vi "updateNVYPartsSerialNo.vi"() -> ()   [LabVIEW 2012]
uses:
  <vilib>/addons/database/Connection.llb/DB Tools Open Connec (Path).vi
  <vilib>/addons/database/Connection.llb/Conn Execute.vi
  <vilib>/addons/database/Recordset.llb/Rec Fetch String Data (R).vi
  <vilib>/addons/database/Recordset.llb/Rec Destroy - Connection.vi
  <vilib>/addons/database/Recordset.llb/Rec Fetch Recordset Data (R).vi
  <vilib>/addons/database/_DB Variant To Data/Database Variant To Data.xnode
  <vilib>/addons/database/NI_Database_API.lvlib
panel:
  out "date/time string 5":string
  out "data 10":string
  out "s? t:f 5":i32
  out "recordset data 5":variant[][](array[variant])
  out "error out 8":errorcluster
  out "error out 7":errorcluster
  out "data 9":string
  out "concatenated string 5":string
  out "x+y 5":i32
  out "date/time string 4":string
  out "data 8":string
  out "s? t:f 4":i32
  out "recordset data 4":variant[][](array[variant])
  out "error out 6":errorcluster
  out "error out 5":errorcluster
  out "data 7":string
  out "concatenated string 4":string
  out "x+y 4":i32
  out "error out 4":errorcluster
  out "date/time string 3":string
  out "data 6":string
  out "s? t:f 3":i32
  out "recordset data 3":variant[][](array[variant])
  out "error out 3":errorcluster
  out "data 5":string
  out "concatenated string 3":string
  out "x+y 3":i32
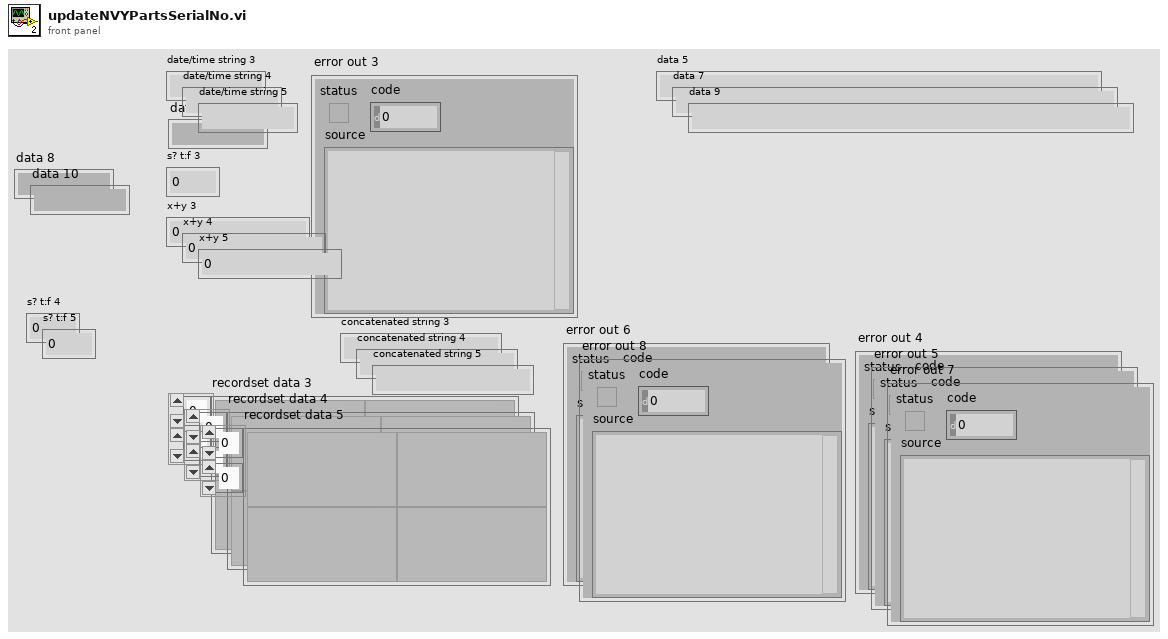
[diagram p1: front panel]
types:
  T1 = typedef "NI_Database_API.lvlib/Conn ObjectReference.ctl" = refnum<k1>
  T2 = typedef "NI_Database_API.lvlib/Rec ObjectReference.ctl" = refnum<k1>
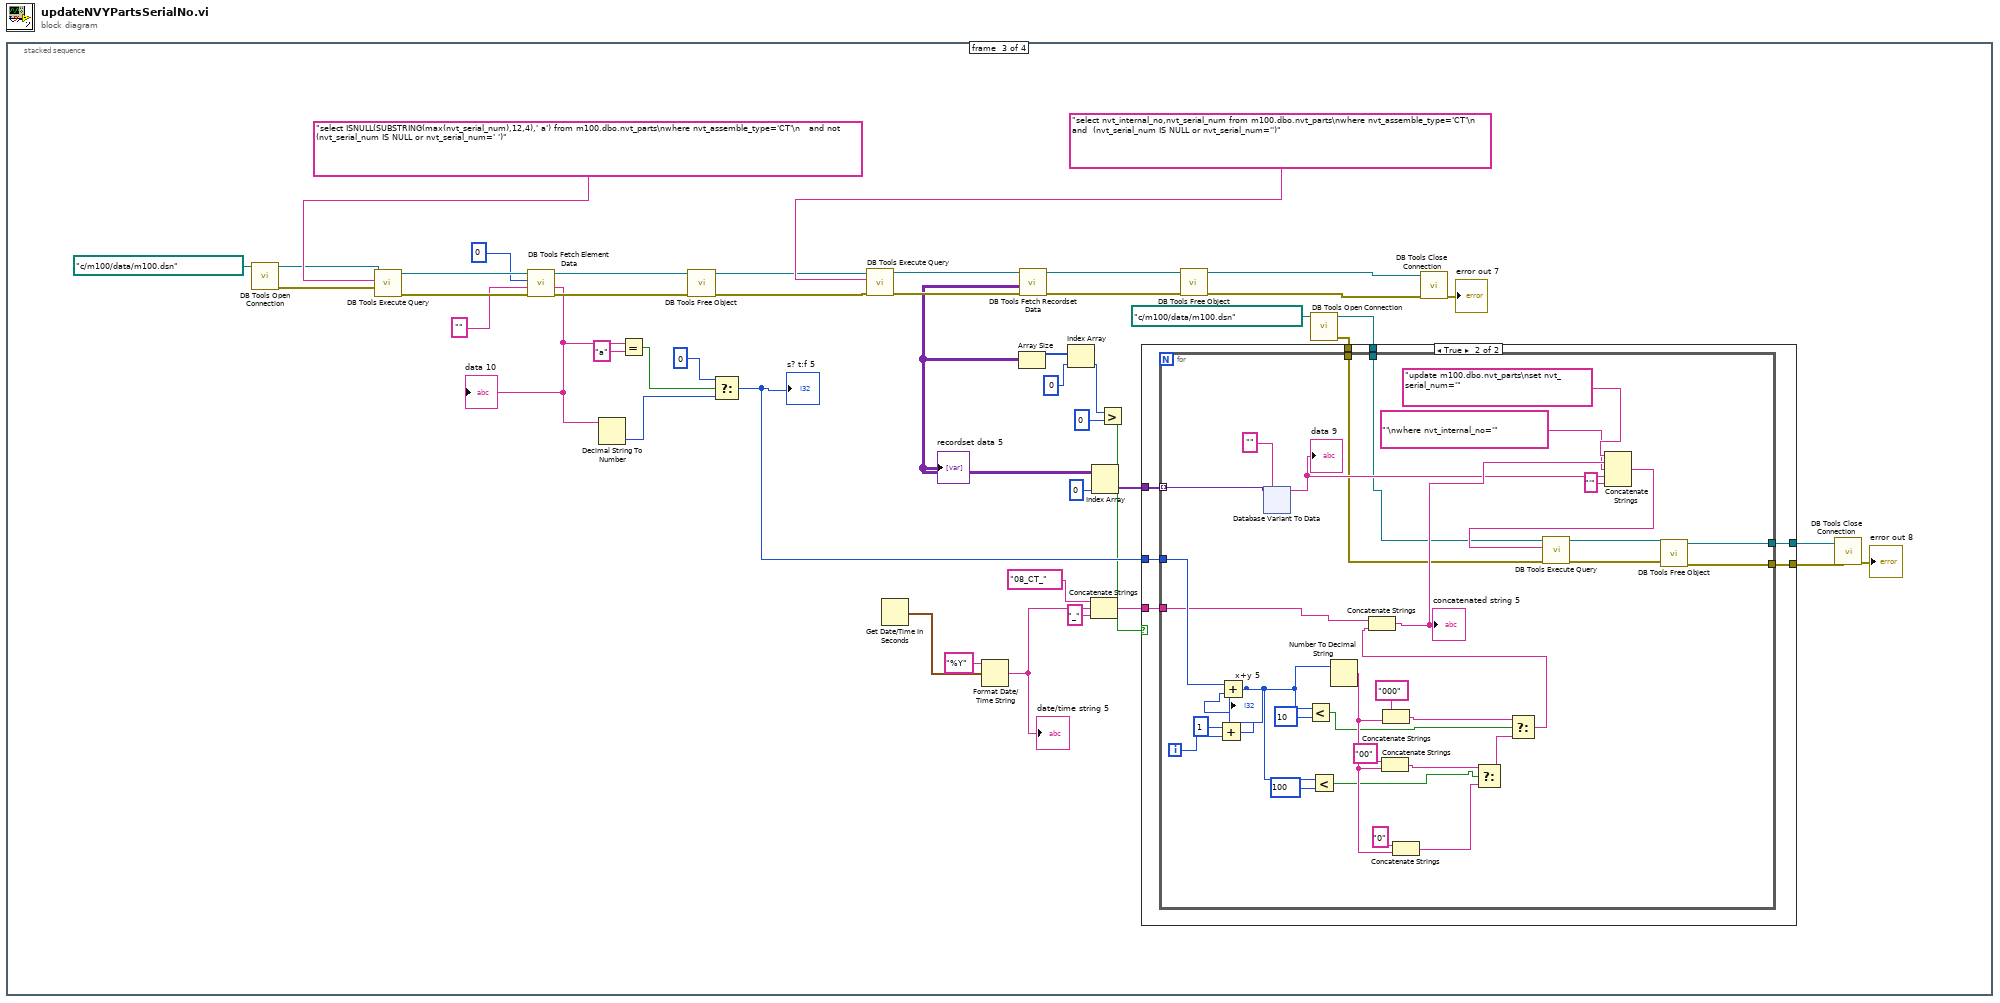
[diagram p0: block diagram]
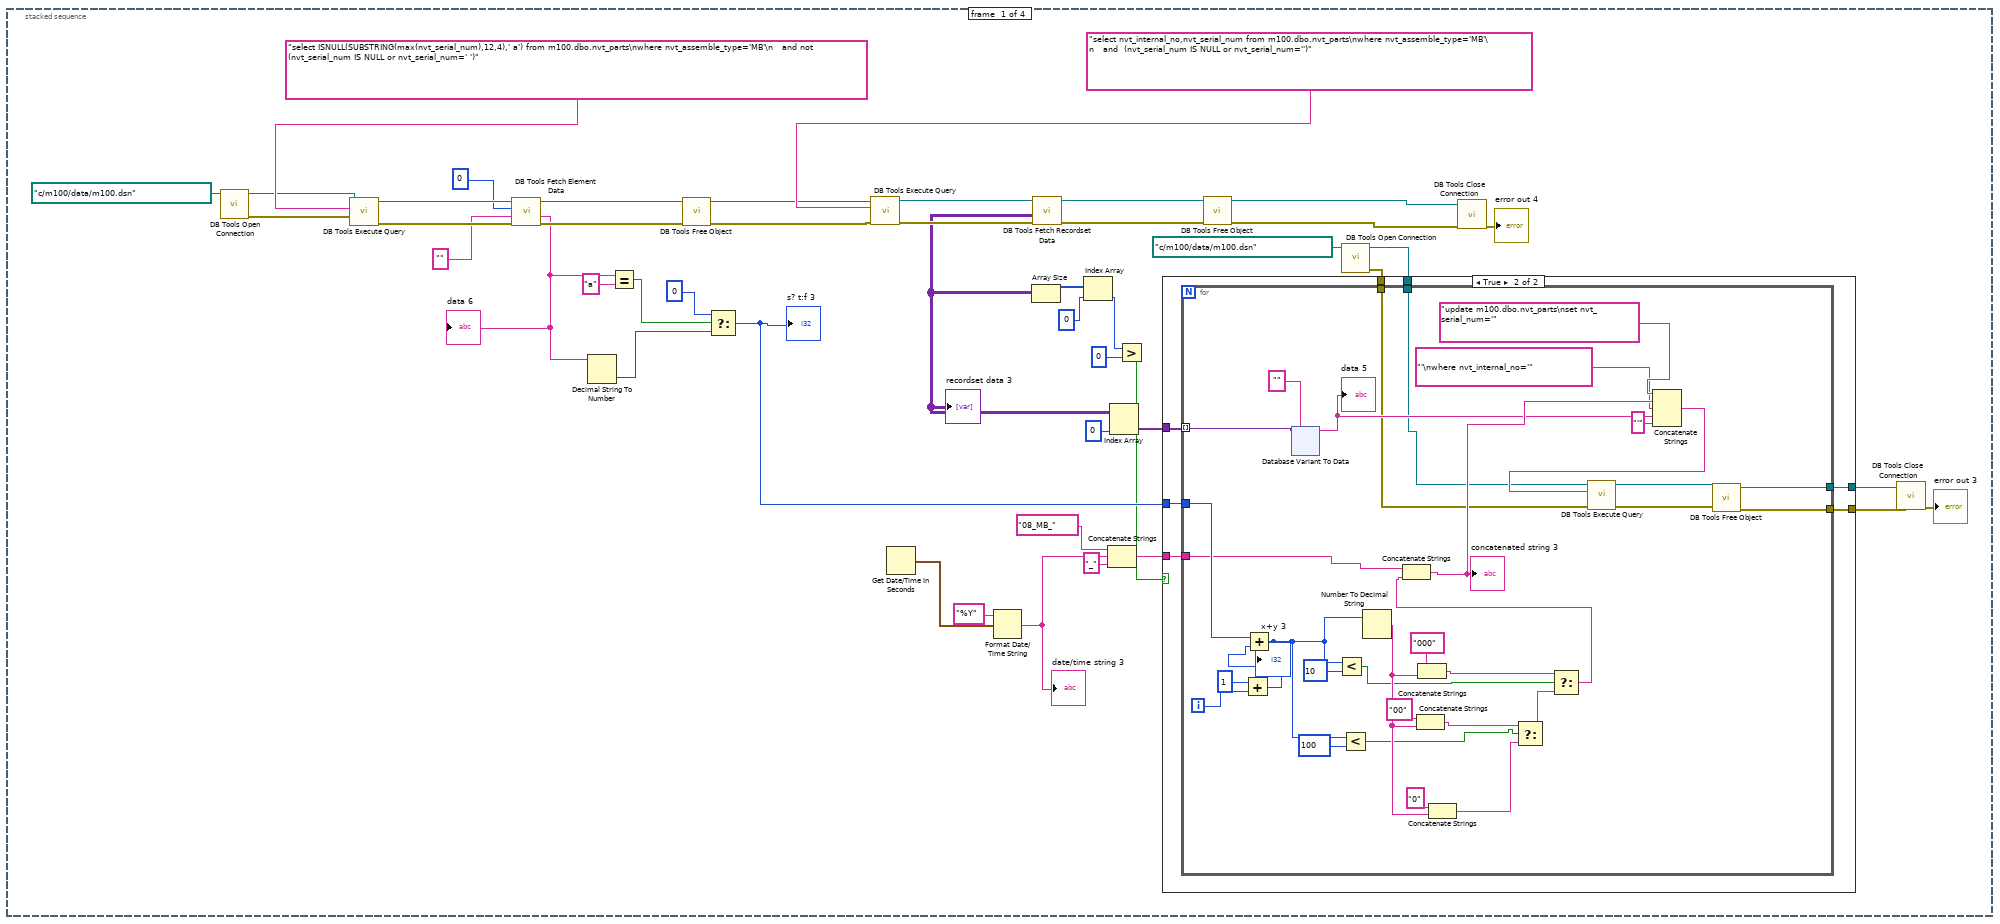
[diagram p2: hidden frame]
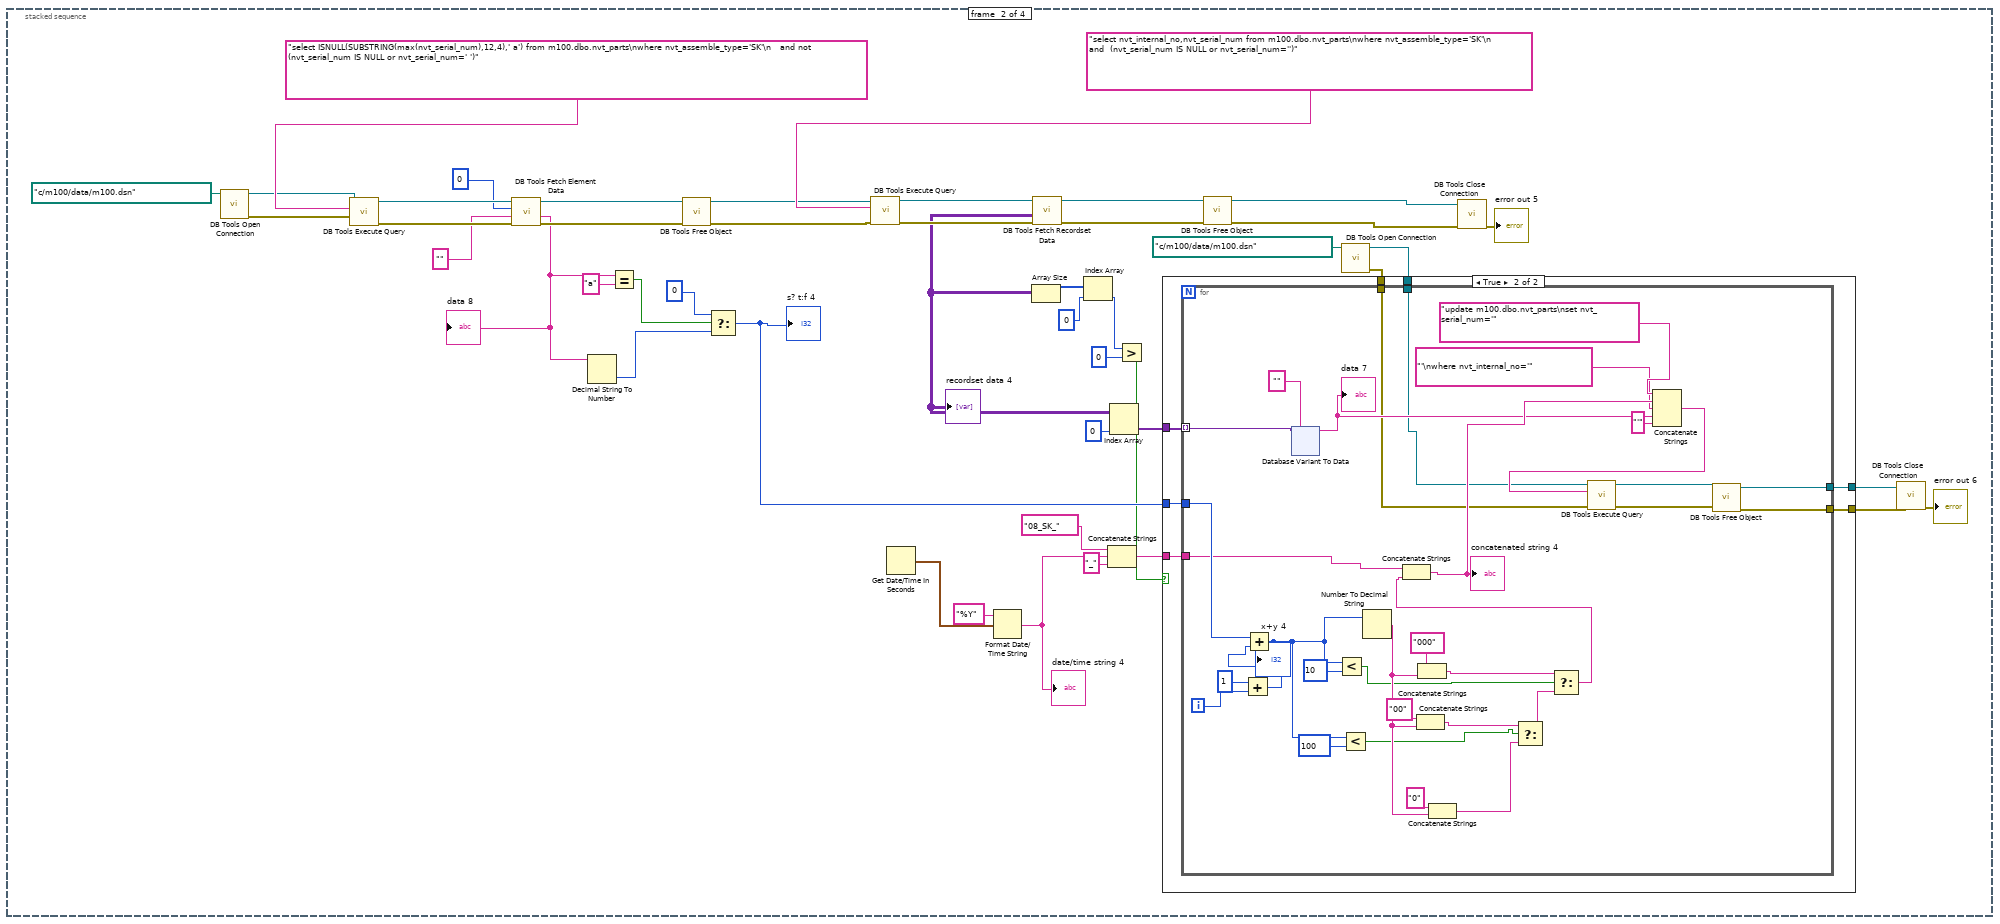
[diagram p4: hidden frame]
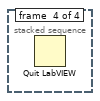
[diagram p7: hidden frame]
diagram:
  n1 = stacked-sequence {
    frame #0 {
      n2 = call-poly <vilib>:"DB Tools Open Connection.vi"("connection information"=path "c:/m100/data/m100.dsn") -> ("error out"=w28:errorcluster, "connection reference"=w29:T1)  [unwired: 7 in]
      n3 = call-poly <vilib>:"DB Tools Execute Query.vi"("error in (no error)"=w28, "SQL query"="select ISNULL(SUBSTRING(max(nvt_serial_num),12,4),' a') from m100.dbo.nvt_parts\nwhere nvt_assemble_type='MB'\n   and not (nvt_serial_num IS NULL or nvt_serial_num=' ')", "connection reference"=w29) -> ("error out"=w32:errorcluster, "recordset reference"=w34:T2)  [unwired: 5 in]
      n4 = call-poly <vilib>:"DB Tools Fetch Element Data.vi"("error in (no error)"=w32, "type"="", "column index"=0, "recordset reference"=w34) -> ("error out"=w31:errorcluster, "data"=w20:string, "recordset reference out"=w33:T2)  [unwired: 3 in]
      "data 6" <- w20
      n5 = Decimal String To Number(string=w20) -> (number=w19:i32)  [unwired: 2 in, 1 out]
      n6 = Equal?(x=w20, y="a") -> (x = y?=w22:bool)
      n7 = call-poly <vilib>:"DB Tools Free Object.vi"("error in (no error)"=w31, "recordset reference"=w33) -> ("error out"=w26:errorcluster, "connection reference"=w27:T1)  [unwired: 8 in]
      n8 = Select(t=0, s=w22, f=w19) -> (s? t:f=w16:i32)
      "s? t:f 3" <- w16
      n9 = call-poly <vilib>:"DB Tools Execute Query.vi"("error in (no error)"=w26, "SQL query"="select nvt_internal_no,nvt_serial_num from m100.dbo.nvt_parts\nwhere nvt_assemble_type='MB'\n   and  (nvt_serial_num IS NULL or nvt_serial_num='')", "connection reference"=w27) -> ("error out"=w44:errorcluster, "recordset reference"=w46:T2)  [unwired: 5 in]
      n10 = Get Date/Time In Seconds() -> (seconds since 1Jan1904=w38:timestamp)
      n11 = Format Date/Time String(time format string (%c)="%Y", seconds (now)=w38) -> (date/time string=w35:string)  [unwired: 1 in]
      "date/time string 3" <- w35
      n12 = call-poly <vilib>:"DB Tools Fetch Recordset Data.vi"("error in (no error)"=w44, "recordset reference"=w46) -> ("error out"=w43:errorcluster, "recordset data"=w14:variant[][], "recordset reference out"=w45:T2)  [unwired: 3 in]
      "recordset data 3" <- w14
      n13 = Array Size(array=w14) -> (size(s)=w13:i32[])
      n14 = Index Array(array=w13, index=0) -> (element=w12:i32)
      n15 = Concatenate Strings("08_MB_" ("string"), w35, "_" ("string")) -> (w17:string)
      n16 = Index Array(array=w14, index (col)=0 ("disabled index (col)")) -> (element=w40:variant[])  [unwired: 1 in]
      n17 = Greater?(x=w12, y=0) -> (0:w1:bool)
      n18 = call-poly <vilib>:"DB Tools Free Object.vi"("error in (no error)"=w43, "recordset reference"=w45) -> ("error out"=w5:errorcluster, "connection reference"=w6:T1)  [unwired: 8 in]
      n19 = call-poly <vilib>:"DB Tools Open Connection.vi"("connection information"=path "c:/m100/data/m100.dsn") -> ("error out"=w3:errorcluster, "connection reference"=w2:T1)  [unwired: 7 in]
      n20 = case shown="True" w1 {
        tunnel: w40 -> [_ w55]
        tunnel: w17 -> [_ w54]
        tunnel: w16 -> [_ w53]
        tunnel: [w48 w52] -> w9
        tunnel: [w47 w51] -> w8
        tunnel: w3 -> [w47 w50]
        tunnel: w2 -> [w48 w49]
        frame False {
        }
        frame True {
          n21 = for {
            tunnel: w55 -> [w88] mode=indexing
            tunnel: w54 -> [w85]
            tunnel: w53 -> [w86]
            tunnel: w49 -> [w61]
            tunnel: w50 -> [w60]
            tunnel: [w58] -> w52
            tunnel: [w56] -> w51
            i -> [w84]
            n22 = Add(x=1, y=w84) -> (x+y=w82:i32)
            n23 = Add(x=w86, y=w82) -> (x+y=w78:i32)
            "x+y 3" <- w78
            n24 = xnode "Database Variant To Data"("database variant"=w88, "type"="") -> ("data"=w64:string)  [unwired: 1 in, 1 out]
            "data 5" <- w64
            n25 = Less?(x=w78, y=10) -> (x < y?=w74:bool)
            n26 = Less?(x=w78, y=100) -> (x < y?=w72:bool)
            n27 = Number To Decimal String(number=w78) -> (decimal integer string=w75:string)  [unwired: 1 in]
            n28 = Concatenate Strings("00" ("string"), w75) -> (w71:string)
            n29 = Concatenate Strings("000" ("string"), w75) -> (w73:string)
            n30 = Concatenate Strings("0" ("string"), w75) -> (w69:string)
            n31 = Select(t=w71, s=w72, f=w69) -> (s? t:f=w70:string)
            n32 = Select(t=w73, s=w74, f=w70) -> (s? t:f=w68:string)
            n33 = Concatenate Strings(w85, w68) -> (w66:string)
            "concatenated string 3" <- w66
            n34 = Concatenate Strings("update m100.dbo.nvt_parts\nset nvt_serial_num='", w66, "'\nwhere nvt_internal_no='" ("string"), w64, "'" ("string")) -> (w62:string)
            n35 = call-poly <vilib>:"DB Tools Execute Query.vi"("error in (no error)"=w60, "SQL query"=w62, "connection reference"=w61) -> ("error out"=w57:errorcluster, "recordset reference"=w59:T2)  [unwired: 5 in]
            n36 = call-poly <vilib>:"DB Tools Free Object.vi"("error in (no error)"=w57, "recordset reference"=w59) -> ("error out"=w56:errorcluster, "connection reference"=w58:T1)  [unwired: 8 in]
          }
        }
      }
      n37 = call <vilib>:"DB Tools Close Connection.vi"("error in (no error)"=w5, "connection reference"=w6) -> ("error out"=→"error out 4":errorcluster)  [unwired: 5 in]
      n38 = call <vilib>:"DB Tools Close Connection.vi"("error in (no error)"=w8, "connection reference"=w9) -> ("error out"=→"error out 3":errorcluster)  [unwired: 5 in]
    }
    frame #1 {
      n39 = call-poly <vilib>:"DB Tools Open Connection.vi"("connection information"=path "c:/m100/data/m100.dsn") -> ("error out"=w148:errorcluster, "connection reference"=w149:T1)  [unwired: 7 in]
      n40 = call-poly <vilib>:"DB Tools Execute Query.vi"("error in (no error)"=w148, "SQL query"="select ISNULL(SUBSTRING(max(nvt_serial_num),12,4),' a') from m100.dbo.nvt_parts\nwhere nvt_assemble_type='SK'\n   and not (nvt_serial_num IS NULL or nvt_serial_num=' ')", "connection reference"=w149) -> ("error out"=w152:errorcluster, "recordset reference"=w154:T2)  [unwired: 5 in]
      n41 = call-poly <vilib>:"DB Tools Fetch Element Data.vi"("error in (no error)"=w152, "type"="", "column index"=0, "recordset reference"=w154) -> ("error out"=w151:errorcluster, "data"=w140:string, "recordset reference out"=w153:T2)  [unwired: 3 in]
      "data 8" <- w140
      n42 = Decimal String To Number(string=w140) -> (number=w139:i32)  [unwired: 2 in, 1 out]
      n43 = Equal?(x=w140, y="a") -> (x = y?=w142:bool)
      n44 = call-poly <vilib>:"DB Tools Free Object.vi"("error in (no error)"=w151, "recordset reference"=w153) -> ("error out"=w146:errorcluster, "connection reference"=w147:T1)  [unwired: 8 in]
      n45 = Select(t=0, s=w142, f=w139) -> (s? t:f=w136:i32)
      "s? t:f 4" <- w136
      n46 = call-poly <vilib>:"DB Tools Execute Query.vi"("error in (no error)"=w146, "SQL query"="select nvt_internal_no,nvt_serial_num from m100.dbo.nvt_parts\nwhere nvt_assemble_type='SK'\n   and  (nvt_serial_num IS NULL or nvt_serial_num='')", "connection reference"=w147) -> ("error out"=w164:errorcluster, "recordset reference"=w166:T2)  [unwired: 5 in]
      n47 = Get Date/Time In Seconds() -> (seconds since 1Jan1904=w158:timestamp)
      n48 = Format Date/Time String(time format string (%c)="%Y", seconds (now)=w158) -> (date/time string=w155:string)  [unwired: 1 in]
      "date/time string 4" <- w155
      n49 = call-poly <vilib>:"DB Tools Fetch Recordset Data.vi"("error in (no error)"=w164, "recordset reference"=w166) -> ("error out"=w163:errorcluster, "recordset data"=w134:variant[][], "recordset reference out"=w165:T2)  [unwired: 3 in]
      "recordset data 4" <- w134
      n50 = Array Size(array=w134) -> (size(s)=w133:i32[])
      n51 = Index Array(array=w133, index=0) -> (element=w132:i32)
      n52 = Concatenate Strings("08_SK_" ("string"), w155, "_" ("string")) -> (w137:string)
      n53 = Index Array(array=w134, index (col)=0 ("disabled index (col)")) -> (element=w160:variant[])  [unwired: 1 in]
      n54 = Greater?(x=w132, y=0) -> (0:w121:bool)
      n55 = call-poly <vilib>:"DB Tools Free Object.vi"("error in (no error)"=w163, "recordset reference"=w165) -> ("error out"=w125:errorcluster, "connection reference"=w126:T1)  [unwired: 8 in]
      n56 = call-poly <vilib>:"DB Tools Open Connection.vi"("connection information"=path "c:/m100/data/m100.dsn") -> ("error out"=w123:errorcluster, "connection reference"=w122:T1)  [unwired: 7 in]
      n57 = case shown="True" w121 {
        tunnel: w160 -> [_ w175]
        tunnel: w137 -> [_ w174]
        tunnel: w136 -> [_ w173]
        tunnel: [w168 w172] -> w129
        tunnel: [w167 w171] -> w128
        tunnel: w123 -> [w167 w170]
        tunnel: w122 -> [w168 w169]
        frame False {
        }
        frame True {
          n58 = for {
            tunnel: w175 -> [w208] mode=indexing
            tunnel: w174 -> [w205]
            tunnel: w173 -> [w206]
            tunnel: w169 -> [w181]
            tunnel: w170 -> [w180]
            tunnel: [w178] -> w172
            tunnel: [w176] -> w171
            i -> [w204]
            n59 = Add(x=1, y=w204) -> (x+y=w202:i32)
            n60 = Add(x=w206, y=w202) -> (x+y=w198:i32)
            "x+y 4" <- w198
            n61 = xnode "Database Variant To Data"("database variant"=w208, "type"="") -> ("data"=w184:string)  [unwired: 1 in, 1 out]
            "data 7" <- w184
            n62 = Less?(x=w198, y=10) -> (x < y?=w194:bool)
            n63 = Less?(x=w198, y=100) -> (x < y?=w192:bool)
            n64 = Number To Decimal String(number=w198) -> (decimal integer string=w195:string)  [unwired: 1 in]
            n65 = Concatenate Strings("00" ("string"), w195) -> (w191:string)
            n66 = Concatenate Strings("000" ("string"), w195) -> (w193:string)
            n67 = Concatenate Strings("0" ("string"), w195) -> (w189:string)
            n68 = Select(t=w191, s=w192, f=w189) -> (s? t:f=w190:string)
            n69 = Select(t=w193, s=w194, f=w190) -> (s? t:f=w188:string)
            n70 = Concatenate Strings(w205, w188) -> (w186:string)
            "concatenated string 4" <- w186
            n71 = Concatenate Strings("update m100.dbo.nvt_parts\nset nvt_serial_num='", w186, "'\nwhere nvt_internal_no='" ("string"), w184, "'" ("string")) -> (w182:string)
            n72 = call-poly <vilib>:"DB Tools Execute Query.vi"("error in (no error)"=w180, "SQL query"=w182, "connection reference"=w181) -> ("error out"=w177:errorcluster, "recordset reference"=w179:T2)  [unwired: 5 in]
            n73 = call-poly <vilib>:"DB Tools Free Object.vi"("error in (no error)"=w177, "recordset reference"=w179) -> ("error out"=w176:errorcluster, "connection reference"=w178:T1)  [unwired: 8 in]
          }
        }
      }
      n74 = call <vilib>:"DB Tools Close Connection.vi"("error in (no error)"=w125, "connection reference"=w126) -> ("error out"=→"error out 5":errorcluster)  [unwired: 5 in]
      n75 = call <vilib>:"DB Tools Close Connection.vi"("error in (no error)"=w128, "connection reference"=w129) -> ("error out"=→"error out 6":errorcluster)  [unwired: 5 in]
    }
    frame #2 {
      n76 = call-poly <vilib>:"DB Tools Open Connection.vi"("connection information"=path "c:/m100/data/m100.dsn") -> ("error out"=w268:errorcluster, "connection reference"=w269:T1)  [unwired: 7 in]
      n77 = call-poly <vilib>:"DB Tools Execute Query.vi"("error in (no error)"=w268, "SQL query"="select ISNULL(SUBSTRING(max(nvt_serial_num),12,4),' a') from m100.dbo.nvt_parts\nwhere nvt_assemble_type='CT'\n   and not (nvt_serial_num IS NULL or nvt_serial_num=' ')", "connection reference"=w269) -> ("error out"=w272:errorcluster, "recordset reference"=w274:T2)  [unwired: 5 in]
      n78 = call-poly <vilib>:"DB Tools Fetch Element Data.vi"("error in (no error)"=w272, "type"="", "column index"=0, "recordset reference"=w274) -> ("error out"=w271:errorcluster, "data"=w260:string, "recordset reference out"=w273:T2)  [unwired: 3 in]
      "data 10" <- w260
      n79 = Decimal String To Number(string=w260) -> (number=w259:i32)  [unwired: 2 in, 1 out]
      n80 = Equal?(x=w260, y="a") -> (x = y?=w262:bool)
      n81 = call-poly <vilib>:"DB Tools Free Object.vi"("error in (no error)"=w271, "recordset reference"=w273) -> ("error out"=w266:errorcluster, "connection reference"=w267:T1)  [unwired: 8 in]
      n82 = Select(t=0, s=w262, f=w259) -> (s? t:f=w256:i32)
      "s? t:f 5" <- w256
      n83 = call-poly <vilib>:"DB Tools Execute Query.vi"("error in (no error)"=w266, "SQL query"="select nvt_internal_no,nvt_serial_num from m100.dbo.nvt_parts\nwhere nvt_assemble_type='CT'\n   and  (nvt_serial_num IS NULL or nvt_serial_num='')", "connection reference"=w267) -> ("error out"=w284:errorcluster, "recordset reference"=w286:T2)  [unwired: 5 in]
      n84 = Get Date/Time In Seconds() -> (seconds since 1Jan1904=w278:timestamp)
      n85 = Format Date/Time String(time format string (%c)="%Y", seconds (now)=w278) -> (date/time string=w275:string)  [unwired: 1 in]
      "date/time string 5" <- w275
      n86 = call-poly <vilib>:"DB Tools Fetch Recordset Data.vi"("error in (no error)"=w284, "recordset reference"=w286) -> ("error out"=w283:errorcluster, "recordset data"=w254:variant[][], "recordset reference out"=w285:T2)  [unwired: 3 in]
      "recordset data 5" <- w254
      n87 = Array Size(array=w254) -> (size(s)=w253:i32[])
      n88 = Index Array(array=w253, index=0) -> (element=w252:i32)
      n89 = Concatenate Strings("08_CT_" ("string"), w275, "_" ("string")) -> (w257:string)
      n90 = Index Array(array=w254, index (col)=0 ("disabled index (col)")) -> (element=w280:variant[])  [unwired: 1 in]
      n91 = Greater?(x=w252, y=0) -> (0:w241:bool)
      n92 = call-poly <vilib>:"DB Tools Free Object.vi"("error in (no error)"=w283, "recordset reference"=w285) -> ("error out"=w245:errorcluster, "connection reference"=w246:T1)  [unwired: 8 in]
      n93 = call-poly <vilib>:"DB Tools Open Connection.vi"("connection information"=path "c:/m100/data/m100.dsn") -> ("error out"=w243:errorcluster, "connection reference"=w242:T1)  [unwired: 7 in]
      n94 = case shown="True" w241 {
        tunnel: w280 -> [_ w295]
        tunnel: w257 -> [_ w294]
        tunnel: w256 -> [_ w293]
        tunnel: [w288 w292] -> w249
        tunnel: [w287 w291] -> w248
        tunnel: w243 -> [w287 w290]
        tunnel: w242 -> [w288 w289]
        frame False {
        }
        frame True {
          n95 = for {
            tunnel: w295 -> [w328] mode=indexing
            tunnel: w294 -> [w325]
            tunnel: w293 -> [w326]
            tunnel: w289 -> [w301]
            tunnel: w290 -> [w300]
            tunnel: [w298] -> w292
            tunnel: [w296] -> w291
            i -> [w324]
            n96 = Add(x=1, y=w324) -> (x+y=w322:i32)
            n97 = Add(x=w326, y=w322) -> (x+y=w318:i32)
            "x+y 5" <- w318
            n98 = xnode "Database Variant To Data"("database variant"=w328, "type"="") -> ("data"=w304:string)  [unwired: 1 in, 1 out]
            "data 9" <- w304
            n99 = Less?(x=w318, y=10) -> (x < y?=w314:bool)
            n100 = Less?(x=w318, y=100) -> (x < y?=w312:bool)
            n101 = Number To Decimal String(number=w318) -> (decimal integer string=w315:string)  [unwired: 1 in]
            n102 = Concatenate Strings("00" ("string"), w315) -> (w311:string)
            n103 = Concatenate Strings("000" ("string"), w315) -> (w313:string)
            n104 = Concatenate Strings("0" ("string"), w315) -> (w309:string)
            n105 = Select(t=w311, s=w312, f=w309) -> (s? t:f=w310:string)
            n106 = Select(t=w313, s=w314, f=w310) -> (s? t:f=w308:string)
            n107 = Concatenate Strings(w325, w308) -> (w306:string)
            "concatenated string 5" <- w306
            n108 = Concatenate Strings("update m100.dbo.nvt_parts\nset nvt_serial_num='", w306, "'\nwhere nvt_internal_no='" ("string"), w304, "'" ("string")) -> (w302:string)
            n109 = call-poly <vilib>:"DB Tools Execute Query.vi"("error in (no error)"=w300, "SQL query"=w302, "connection reference"=w301) -> ("error out"=w297:errorcluster, "recordset reference"=w299:T2)  [unwired: 5 in]
            n110 = call-poly <vilib>:"DB Tools Free Object.vi"("error in (no error)"=w297, "recordset reference"=w299) -> ("error out"=w296:errorcluster, "connection reference"=w298:T1)  [unwired: 8 in]
          }
        }
      }
      n111 = call <vilib>:"DB Tools Close Connection.vi"("error in (no error)"=w245, "connection reference"=w246) -> ("error out"=→"error out 7":errorcluster)  [unwired: 5 in]
      n112 = call <vilib>:"DB Tools Close Connection.vi"("error in (no error)"=w248, "connection reference"=w249) -> ("error out"=→"error out 8":errorcluster)  [unwired: 5 in]
    }
    frame #3 {
      n113 = Quit LabVIEW() -> ()  [unwired: 1 in]
    }
  }
